vi "Trial Distance Graph Accumulator.vi"(7 "Start Test":bool, 10 "Seconds of history:":dbl=20.0 format="%.1f", 11 "Period(ms)":i32=250) -> (0 "LatestPoint":cluster{"X":dbl, "Y":dbl}, 1 "cur_trial_distance":dbl, 3 "Graph OUT":cluster{"X":dbl, "Y":dbl}[](array[cluster]))   [LabVIEW 2018]
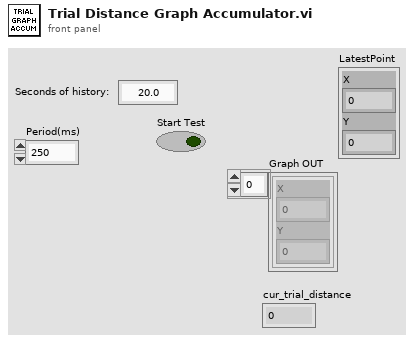
[diagram p1: front panel]
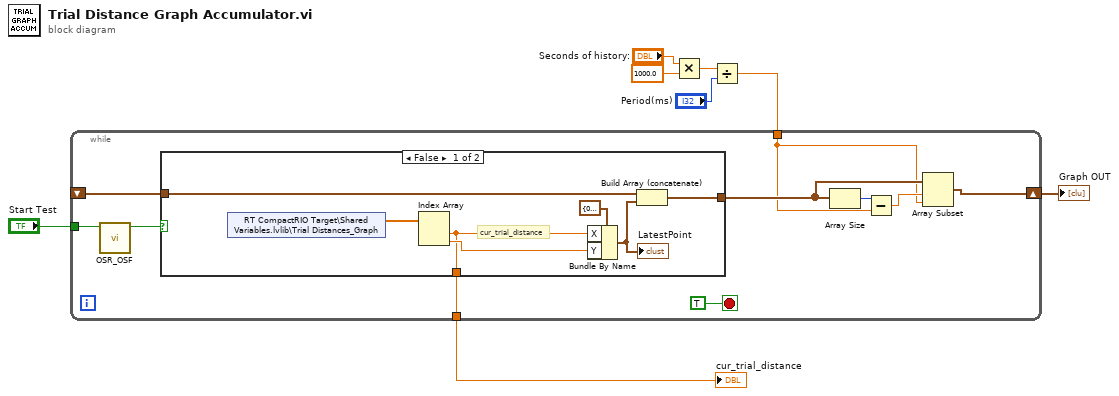
[diagram p0: block diagram]
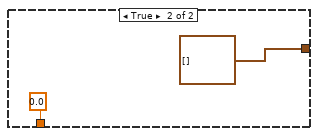
[diagram p2: hidden frame]
diagram:
  n1 = Multiply(x="Seconds of history:", y=1000.0) -> (x*y=w4:dbl)
  n2 = Divide(x=w4, y="Period(ms)") -> (x/y=w1:dbl)
  n3 = while {
    tunnel: "Start Test" -> [w10]
    tunnel: [w17] -> w6
    shift-right: [w12] -> w7
    shift-left: _ -> [w18]
    tunnel: w1 -> [w11]
    stop <- TRUE stop-if-true
    n4 = call "OSR_OSF.vi"("BOOL"=w10) -> ("OSR"=w9:bool)  [unwired: 9 in, 1 out]
    n5 = case shown="False" w9 {
      tunnel: w18 -> [w21 _]
      tunnel: [w20 cluster{"X":dbl, "Y":dbl}[] []] -> w13
      tunnel: [w19 0.0 ("Numeric")] -> w17
      frame False {
        # "cur_trial_distance"
        n6 = shared-variable "RT CompactRIO Target\\Shared Variables.lvlib\\Trial Distances_Graph"() -> (w23:dbl[])  [unwired: 1 in, 1 out]
        n7 = Index Array(array=w23) -> (element #1=w19:dbl, element #2=w22:dbl)  [unwired: 2 in]
        n8 = Bundle By Name(cluster=cluster{"X":dbl, "Y":dbl} {"X"=0.0, "Y"=0.0}, "X"=w19, "Y"=w22) -> (w25:cluster{"X":dbl, "Y":dbl})
        "LatestPoint" <- w25
        n9 = Build Array (concatenate)(w21, w25) -> (w20:cluster{"X":dbl, "Y":dbl}[])
      }
      frame True {
      }
    }
    n10 = Array Size(array=w13) -> (size(s)=w14:i32)
    n11 = Subtract(x=w14, y=w11) -> (x-y=w15:dbl)
    n12 = Array Subset(array=w13, index=w15, length=w11) -> (w12:cluster{"X":dbl, "Y":dbl}[])
  }
  "Graph OUT" <- w7
  "cur_trial_distance" <- w6
